vi "UsrProfiles-Rename profile core.vi"(6 "New user":bool, 8 "error in (no error)":errorcluster, 11 "Source profile's filepath":path) -> (0 "error out":errorcluster, 1 "Cancelled":bool, 2 "New profile name":string, 3 "Filepath of profile to be created":path)   [LabVIEW 2020]
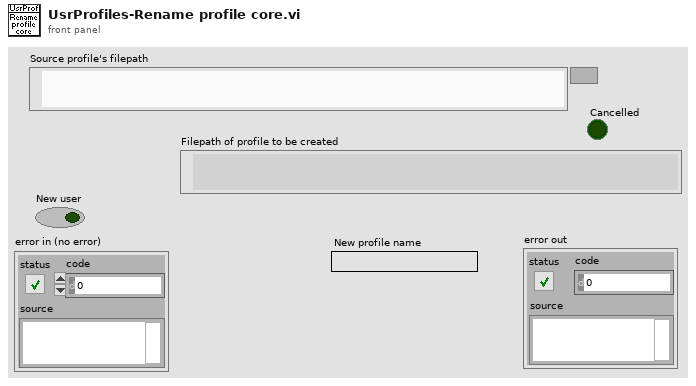
[diagram p1: front panel]
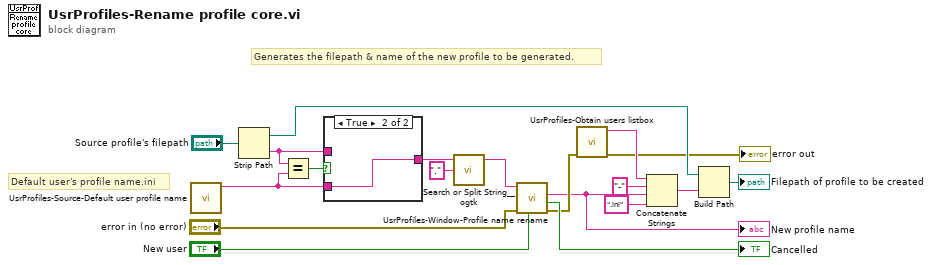
[diagram p0: block diagram]
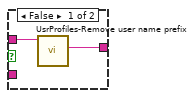
[diagram p2: hidden frame]
diagram:
  # "Default user's profile name.ini"
  # "Generates the filepath & name of the new profile to be generated."
  n1 = call "UsrProfiles-Source-Default user profile name.vi"() -> ("Default user's profile file name & extension"=w1:string)  [unwired: 11 in]
  n2 = Strip Path(path="Source profile's filepath") -> (stripped path=w19:path, name=w15:string)
  n3 = Equal?(x=w15, y=w1) -> (x = y?=w14:bool)
  n4 = case shown="True" w14 {
    tunnel: w1 -> [_ w22]
    tunnel: w15 -> [w21 _]
    tunnel: [w20 w22] -> w10
    frame False {
      n5 = call "UsrProfiles-Remove user name prefix.vi"("Profile name (full)"=w21) -> ("Profile name (user removed)"=w20:string)  [unwired: 10 in]
    }
    frame True {
    }
  }
  n6 = call <userlib>:"Search or Split String__ogtk.vi"("search string/char (-)"=".", "string"=w10) -> ("substring before match"=w11:string)  [unwired: 1 in, 2 out]
  n7 = call "UsrProfiles-Window-Profile name rename.vi"("New user? (F)"="New user", "error in (no error)"="error in (no error)", "Profile name"=w11) -> ("error out"=w5:errorcluster, "Cancelled (Left button pressed)"=→"Cancelled":bool, "New profile name"=w2:string)  [unwired: 6 in]
  "New profile name" <- w2
  n8 = call "UsrProfiles-Obtain users listbox.vi"("error in (no error)"=w5) -> ("error out"=→"error out":errorcluster, "Selected user's name"=w6:string)  [unwired: 7 in, 2 out]
  n9 = Concatenate Strings(w6, "-" ("string"), w2, ".ini" ("string")) -> (w17:string)
  n10 = Build Path(base path=w19, name or relative path=w17) -> (appended path=→"Filepath of profile to be created":path)
